vi "Butterfly_PullDown RC2.vi"(0 "Semiconductor Module Context":T1, 1 "RFPins":string[](array[string]), 2 "current level":dbl=0.01 format="%_6p", 3 "R Thresholds":dbl[](array[numeric]), 5 "error in (no error)":errorcluster, 7 "Start_v":dbl=10.0 format="%#_13g", 9 "Stop_v":dbl=41.0 format="%#_13g", 11 "Step_v":dbl=1.0) -> (14 "Semiconductor Module Context Out":T1, 19 "error out":errorcluster)   [LabVIEW 2013]
uses:
  <vilib>/NI_TestStand_SemiconductorModule/NI_TestStand_Semiconductor_Module.lvlibp/PinMap/General/SemiconductorModuleContext.ctl
  <instrlib>/niDCPower/nidcpower.llb/niDCPower Wait For Event - Event.ctl
  <vilib>/NI_TestStand_SemiconductorModule/NI_TestStand_Semiconductor_Module.lvlibp/PinMap/DC Power/PinsToNIDCPowerSessions.vi
  <vilib>/NI_TestStand_SemiconductorModule/NI_TestStand_Semiconductor_Module.lvlibp/PinMap/General/Publish/PublishDataDoubleFunctionalTest.vi
  <vilib>/NI_TestStand_SemiconductorModule/NI_TestStand_Semiconductor_Module.lvlibp
panel:
  out "Full R Array":dbl[][][](array[numeric])
  out "step":i32
  out "Instrument Session":refnum<k15>
  out "sites and pins loop iter":i32
  out "Channel List":string
  out "BF values":dbl[](array[numeric])
  out "BF Names":string[](array[string])
  out "R Array":dbl[](array[numeric])
  out "BFSamples":i32
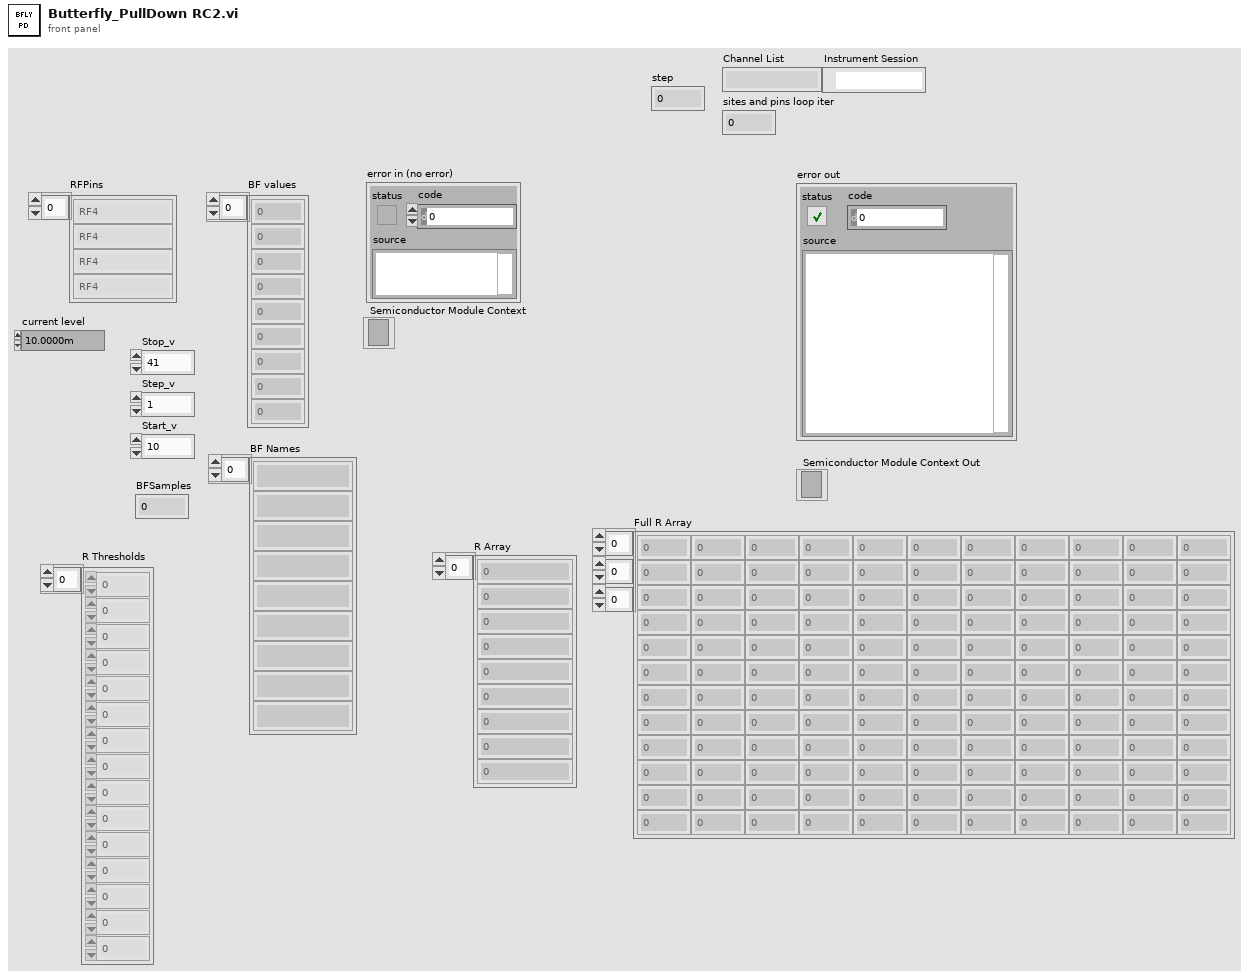
[diagram p1: front panel]
types:
  T1 = typedef "NI_TestStand_Semiconductor_Module.lvlibp/SemiconductorModuleContext.ctl" = refnum<k7>
  T2 = typedef "niDCPower Wait For Event - Event.ctl" = i32
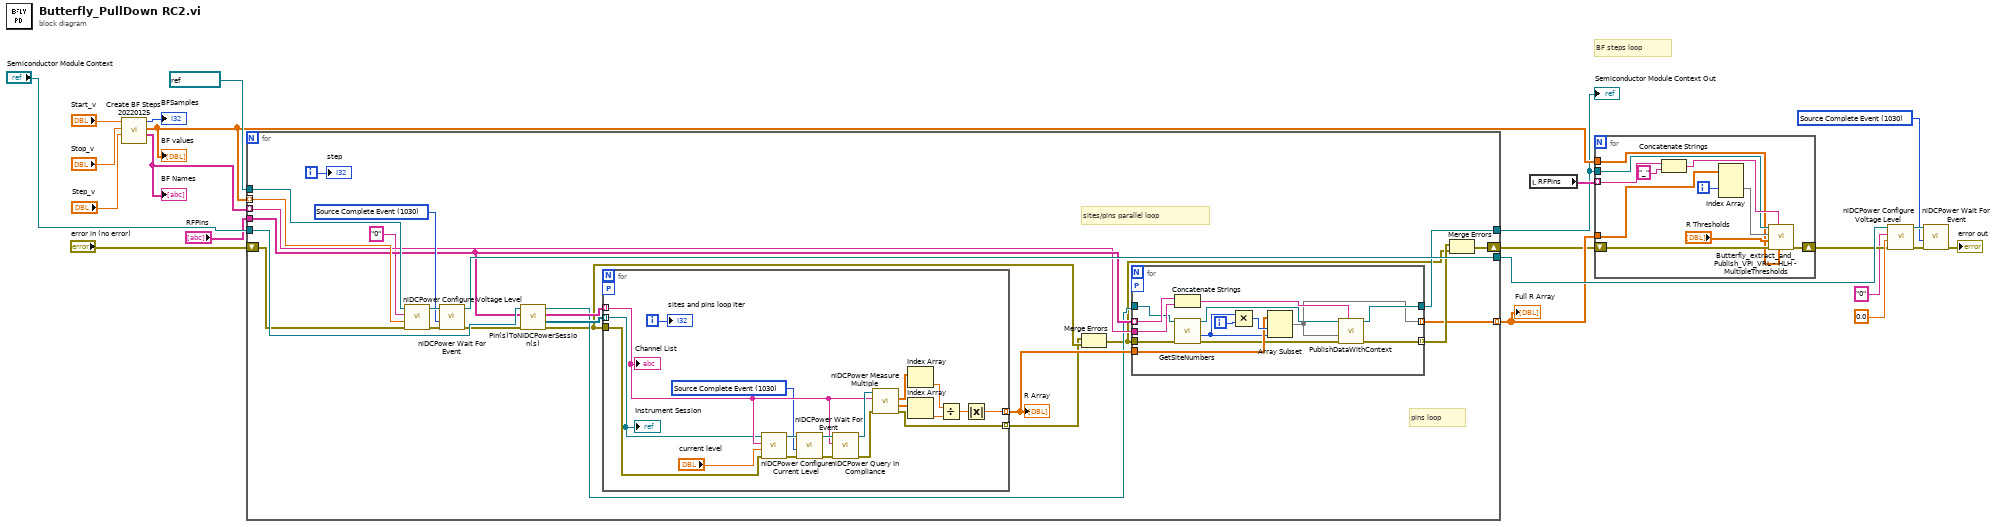
[diagram p0: block diagram]
diagram:
  w10 = T2 1030 items=["Source Complete Event"=1030, "Measure Complete Event"=1031, "Sequence Iteration Complete Event"=1032, "Sequence Engine Done Event"=1033, "Pulse Complete Event"=1051, "Ready For Pulse Trigger Event"=1052] ("event")
  # "BF steps loop"
  n1 = call "Create BF Steps 20220125.vi"("Step_v"="Step_v", "Stop_v"="Stop_v", "Start_v"="Start_v") -> ("BF Names"=w8:string[], "BF values"=w5:dbl[], "BFSamples"=→"BFSamples":i32)  [unwired: 6 in]
  "BF Names" <- w8
  "BF values" <- w5
  n2 = for {
    shift-right: [w27] -> w3
    shift-left: "error in (no error)" -> [w42]
    tunnel: w5 -> [w40] mode=indexing
    tunnel: refnum<k15> "4139_1" ("instrument handle") -> [w39]
    tunnel: [w38] -> w14
    tunnel: "RFPins" -> [w33]
    tunnel: w8 -> [w31] mode=indexing
    tunnel: [w28] -> w6 mode=indexing
    tunnel: "Semiconductor Module Context" -> [w46]
    tunnel: [w30] -> w1
    i -> [w35]
    w44 = T2 1030 items=["Source Complete Event"=1030, "Measure Complete Event"=1031, "Sequence Iteration Complete Event"=1032, "Sequence Engine Done Event"=1033, "Pulse Complete Event"=1051, "Ready For Pulse Trigger Event"=1052] ("event")
    # "pins loop"
    # "sites/pins parallel loop"
    n3 = call <instrlib>:"niDCPower Configure Voltage Level.vi"("error in (no error)"=w42, "voltage level"=w40, "channel name"="0", "instrument handle"=w39) -> ("error out"=w43:errorcluster, "instrument handle out"=w45:refnum<k15>)  [unwired: 6 in]
    n4 = call <instrlib>:"niDCPower Wait For Event.vi"("error in (no error)"=w43, "event"=w44, "instrument handle"=w45) -> ("error out"=w41:errorcluster, "instrument handle out"=w38:refnum<k15>)  [unwired: 7 in]
    n5 = call-poly <vilib>:"Pin(s)ToNIDCPowerSession(s).vi"("error in (no error)"=w41, "Pins"=w33, "Semiconductor Module Context"=w46) -> ("error out"=w25:errorcluster, "Instrument Sessions"=w37:refnum<k15>[], "Channel Lists"=w36:string[], "Semiconductor Module Context Out"=w29:T1)  [unwired: 4 in, 1 out]
    n6 = for {
      tunnel: w36 -> [w66] mode=indexing
      tunnel: w37 -> [w63] mode=indexing
      tunnel: w25 -> [w64]
      tunnel: [w67] -> w32 mode=indexing
      tunnel: [w61] -> w24 mode=indexing
      workers-P: _ -> [_]
      i -> [w62]
      w65 = T2 1030 items=["Source Complete Event"=1030, "Measure Complete Event"=1031, "Sequence Iteration Complete Event"=1032, "Sequence Engine Done Event"=1033, "Pulse Complete Event"=1051, "Ready For Pulse Trigger Event"=1052] ("event")
      n7 = call <instrlib>:"niDCPower Configure Current Level.vi"("error in (no error)"=w64, "current level"="current level", "channel name"=w66, "instrument handle"=w63) -> ("error out"=w75:errorcluster, "instrument handle out"=w74:refnum<k15>)  [unwired: 6 in]
      n8 = call <instrlib>:"niDCPower Wait For Event.vi"("error in (no error)"=w75, "event"=w65, "instrument handle"=w74) -> ("error out"=w79:errorcluster, "instrument handle out"=w78:refnum<k15>)  [unwired: 7 in]
      n9 = call <instrlib>:"niDCPower Query In Compliance.vi"("error in (no error)"=w79, "channel name"=w66, "instrument handle"=w78) -> ("error out"=w76:errorcluster, "instrument handle out"=w77:refnum<k15>)  [unwired: 6 in, 1 out]
      n10 = call <instrlib>:"niDCPower Measure Multiple.vi"("error in (no error)"=w76, "channel name"=w66, "instrument handle"=w77) -> ("error out"=w61:errorcluster, "current measurements"=w68:dbl[], "voltage measurements"=w69:dbl[])  [unwired: 5 in, 1 out]
      n11 = Index Array(array=w69) -> (element=w71:dbl)  [unwired: 1 in]
      n12 = Index Array(array=w68) -> (element=w70:dbl)  [unwired: 1 in]
      n13 = Divide(x=w71, y=w70) -> (x/y=w72:dbl)
      n14 = Absolute Value(x=w72) -> (abs(x)=w67:dbl)
      "Channel List" <- w66
      "sites and pins loop iter" <- w62
      "Instrument Session" <- w63
    }
    "R Array" <- w32
    n15 = Merge Errors(w24, w25) -> (w23:errorcluster)
    n16 = for {
      tunnel: [w55] -> w34 mode=indexing
      tunnel: w33 -> [w59] mode=indexing
      tunnel: w32 -> [w56]
      tunnel: w31 -> [w58]
      tunnel: [w52] -> w28 mode=indexing
      tunnel: w23 -> [w47]
      workers-P: _ -> [_]
      tunnel: w29 -> [w50]
      tunnel: [w53] -> w30
      i -> [w60]
      n17 = Concatenate Strings(w59, w58) -> (w54:string)
      n18 = call <vilib>:"GetSiteNumbers.vi"("error in (no error)"=w47, "Semiconductor Module Context"=w50) -> ("error out"=w51:errorcluster, "Number Of Sites"=w48:i32, "Semiconductor Module Context Out"=w49:T1)  [unwired: 6 in, 1 out]
      n19 = Multiply(x=w48, y=w60) -> (x*y=w57:i32)
      n20 = Array Subset(array=w56, index=w57, length=w48) -> (w52:dbl[])
      n21 = call-poly <vilib>:"PublishDataWithContext.vi"("Published Data Id"=w54, "error in (no error)"=w51, "Data In"=w52, "Semiconductor Module Context"=w49) -> ("error out"=w55:errorcluster, "Semiconductor Module Context Out"=w53:T1)  [unwired: 6 in]
    }
    n22 = Merge Errors(w34, w23) -> (w27:errorcluster)
    "step" <- w35
  }
  "Semiconductor Module Context Out" <- w1
  "Full R Array" <- w6
  n23 = local read "RFPins"() -> (w7:string[])
  n24 = for {
    tunnel: w7 -> [w84] mode=indexing
    tunnel: w6 -> [w89]
    shift-right: [w85] -> w4
    shift-left: w3 -> [w86]
    tunnel: w1 -> [w81]
    tunnel: w5 -> [w80]
    i -> [w90]
    n25 = Concatenate Strings(w84, "_" ("string")) -> (w82:string)
    n26 = Index Array(array=w89, index (dim 1)=w90) -> (element=w87:dbl[][])  [unwired: 2 in]
    n27 = call "Butterfly_extract_and_Publish_VPI_VRL - HLH - MultipleThresholds.vi"("Voltages Array"=w80, "ID Prefix"=w82, "error in (no error)"=w86, "Thresholds"="R Thresholds", "Result Array In"=w87, "Semiconductor Module Context"=w81) -> ("error out"=w85:errorcluster)  [unwired: 5 in]
  }
  n28 = call <instrlib>:"niDCPower Configure Voltage Level.vi"("error in (no error)"=w4, "voltage level"=0.0, "channel name"="0", "instrument handle"=w14) -> ("error out"=w13:errorcluster, "instrument handle out"=w11:refnum<k15>)  [unwired: 6 in]
  n29 = call <instrlib>:"niDCPower Wait For Event.vi"("error in (no error)"=w13, "event"=w10, "instrument handle"=w11) -> ("error out"=→"error out":errorcluster)  [unwired: 7 in, 1 out]
